vi "Query (CryoCon_continuous).vi"(3 "error in (no error)":errorcluster, 4 "write buffer":string, 5 "byte count":u32, 6 "VISA resource name":refnum<visa-resource-name>) -> (0 "error out":errorcluster, 1 "VISA resource name out":refnum<visa-resource-name>, 2 "read buffer":string)   [LabVIEW 2011]
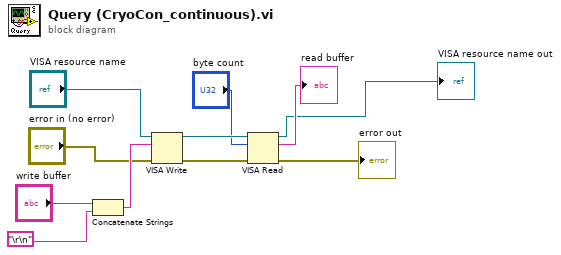
[diagram p0: block diagram]
diagram:
  n1 = Concatenate Strings("write buffer", "\r\n") -> (w9:string)
  n2 = VISA Write(VISA resource name="VISA resource name", write buffer=w9, error in (no error)="error in (no error)") -> (VISA resource name out=w11:refnum<visa-resource-name>, error out=w7:errorcluster)  [unwired: 1 out]
  n3 = VISA Read(VISA resource name=w11, byte count="byte count", error in (no error)=w7) -> (VISA resource name out=→"VISA resource name out":refnum<visa-resource-name>, read buffer=→"read buffer":string, error out=→"error out":errorcluster)  [unwired: 1 out]
